vi "DAQcreateTriggers.vi"() -> ()   [LabVIEW 2020]
uses:
  <vilib>/DAQmx/write.llb/DAQmx Write (Digital Bool 1Line 1Point).vi
  <vilib>/DAQmx/miscellaneous.llb/DAQmx Fill In Error Info.vi
panel:
  out ".not. x?":bool
  in  "stop":bool
  in  "DAQmx Task Name":refnum<k21>
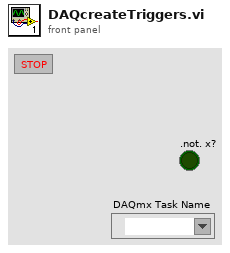
[diagram p1: front panel]
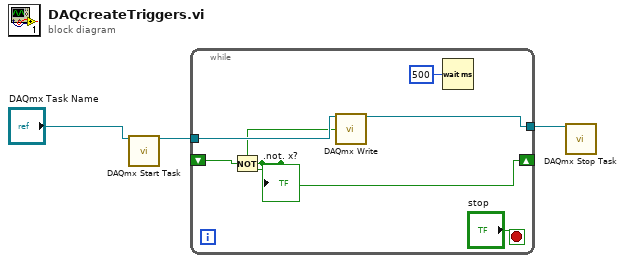
[diagram p0: block diagram]
diagram:
  n1 = call <vilib>:"DAQmx Start Task.vi"("task/channels in"="DAQmx Task Name") -> ("task out"=w2:refnum<k21>)  [unwired: 13 in, 1 out]
  n2 = while {
    tunnel: w2 -> [w8]
    tunnel: [w5] -> w1
    shift-right: [w4] -> _
    shift-left: _ -> [w7]
    stop <- "stop" stop-if-true
    n3 = Not(x=w7) -> (.not. x?=w4:bool)
    ".not. x?" <- w4
    n4 = call-poly <vilib>:"DAQmx Write.vi"("task/channels in"=w8, "data"=w4) -> ("task out"=w5:refnum<k21>)  [unwired: 11 in, 2 out]
    n5 = Wait (ms)(milliseconds to wait=u32 500) -> ()  [unwired: 1 out]
  }
  n6 = call <vilib>:"DAQmx Stop Task.vi"("task/channels in"=w1) -> ()  [unwired: 13 in, 2 out]
